vi "getGoalByName.vi"(7 "Category Name":string, 8 "error in (no error)":errorcluster, 9 "Month":T1, 10 "YYYY":i32, 11 "Account History in":refnum<class "Account History.lvclass">) -> (0 "error out":errorcluster, 2 "Goal":refnum<class "Goal.lvclass">, 3 "Account History out":refnum<class "Account History.lvclass">)   [LabVIEW 2018, in "Account History.lvclass"]
uses:
  Account History.lvclass
  Month.ctl
  Goal/Goal.lvclass
  Category/Category.lvclass
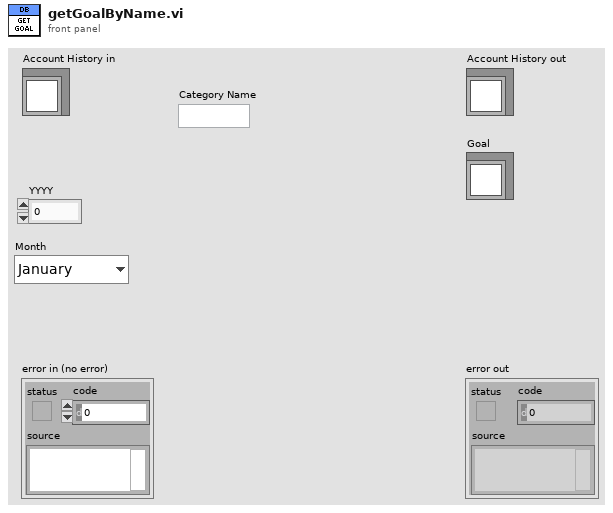
[diagram p1: front panel]
types:
  T1 = typedef "Account History.lvclass/Month.ctl" = enum16{"January", "February", "March", "April", "May", "June", "July", "August", "September", "October", "November", "December"}
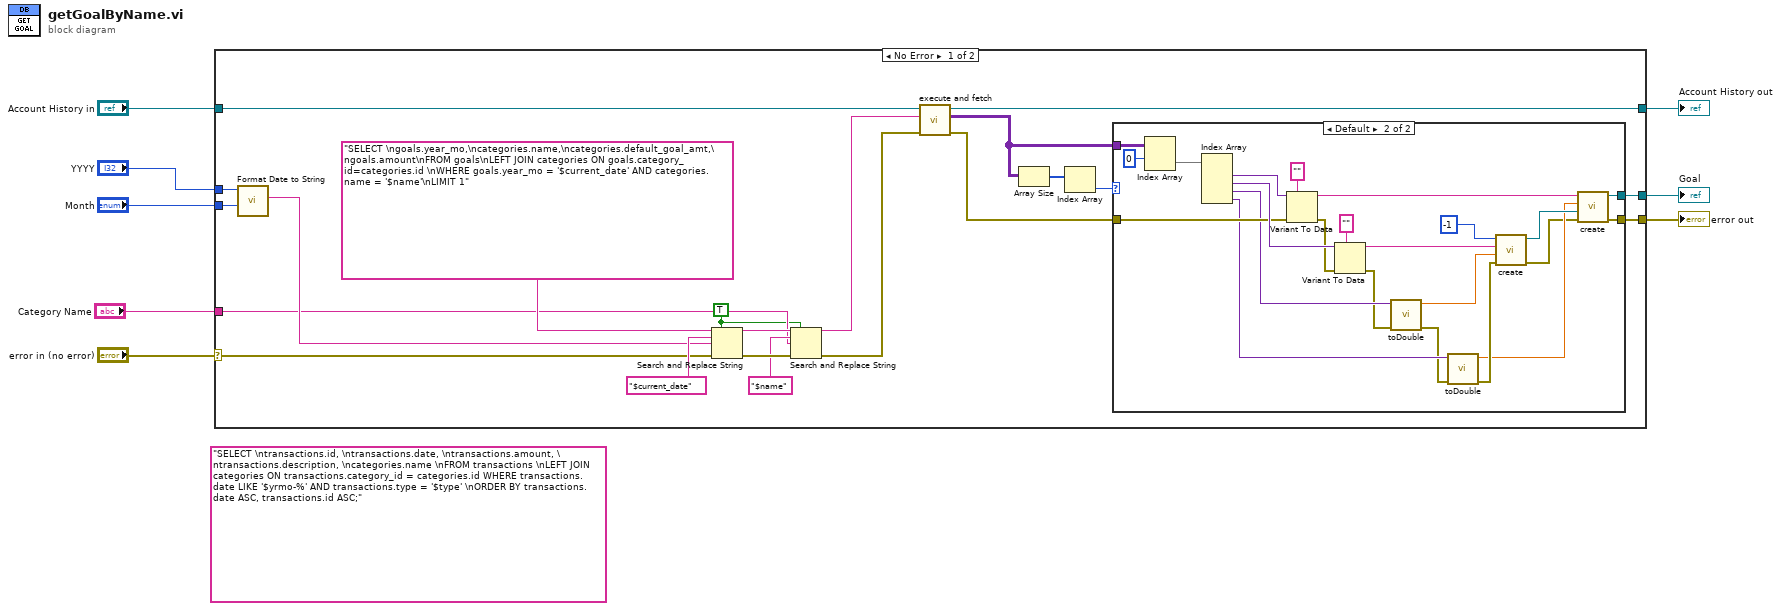
[diagram p0: block diagram]
diagram:
  (unwired) "SELECT \ntransactions.id, \ntransactions.date, \ntransactions.amount, \ntransactions.description, \ncategories.name \nFROM transactions \nLEFT JOIN categories ON transactions.category_id = categories.id WHERE transactions.date LIKE '$yrmo-%' AND transactions.type = '$type' \nORDER BY transactions.date ASC, transactions.id ASC;"
  n1 = case shown="No Error" "error in (no error)" {
    selector: "error in (no error)" -> [w23 w55]
    tunnel: [w14 w55] -> w7
    tunnel: [w26 w54] -> w5
    tunnel: "Account History in" -> [w27 w54]
    tunnel: "YYYY" -> [w29 _]
    tunnel: "Month" -> [w28 _]
    tunnel: "Category Name" -> [w16 _]
    tunnel: [w13 _] -> w1
    frame No Error {
      w15 = TRUE ("replace all? (F)")
      n2 = call "Format Date to String.vi"("Month"=w28, "YYYY"=w29) -> ("Year-Mo"=w22:string)  [unwired: 9 in]
      n3 = Search and Replace String(replace all?=w15, input string="SELECT \ngoals.year_mo,\ncategories.name,\ncategories.default_goal_amt,\ngoals.amount\nFROM goals\nLEFT JOIN categories ON goals.category_id=categories.id \nWHERE goals.year_mo = '$current_date' AND categories.name = '$name'\nLIMIT 1", search string="$current_date", replace string=w22, error in=w23) -> (result string=w20:string, error out=w21:errorcluster)  [unwired: 3 in, 2 out]
      n4 = Search and Replace String(replace all?=w15, input string=w20, search string="$name", replace string=w16, error in=w21) -> (result string=w19:string, error out=w18:errorcluster)  [unwired: 3 in, 2 out]
      n5 = call "execute and fetch.vi"("error in (no error)"=w18, "SQL query"=w19, "Database in"=w27) -> ("error out"=w12:errorcluster, "recordset data"=w11:variant[][], "Database out"=w26:refnum<class "Account History.lvclass">)  [unwired: 5 in, 1 out]
      n6 = Array Size(array=w11) -> (size(s)=w10:i32[])
      n7 = Index Array(array=w10) -> (element=w9:i32)  [unwired: 1 in]
      n8 = case shown="Default" w9 {
        tunnel: [w30 w40] -> w14
        tunnel: [_ w39] -> w13
        tunnel: w12 -> [w30 w38]
        tunnel: w11 -> [_ w31]
        frame 0 {
        }
        frame Default {
          n9 = Index Array(array=w31, index (row)=0) -> (element=w53:variant[])  [unwired: 1 in]
          n10 = Index Array(array=w53) -> (element #1=w52:variant, element #2=w51:variant, element #3=w36:variant, element #4=w37:variant)  [unwired: 4 in]
          n11 = Variant To Data(error in=w38, type="", Variant=w52) -> (data=w49:string, error out=w45:errorcluster)
          n12 = Variant To Data(error in=w45, type="", Variant=w51) -> (data=w47:string, error out=w35:errorcluster)
          n13 = call "toDouble.vi"("error in (no error)"=w35, "Value"=w36) -> ("error out"=w33:errorcluster, "type"=w34:dbl)  [unwired: 8 in]
          n14 = call "toDouble.vi"("error in (no error)"=w33, "Value"=w37) -> ("error out"=w44:errorcluster, "type"=w42:dbl)  [unwired: 8 in]
          n15 = call "create.vi"("error in (no error)"=w44, "Default Goal Amount"=w34, "Name"=w47, "id"=-1) -> ("error out"=w41:errorcluster, "Category out"=w43:refnum<class "Category.lvclass">)  [unwired: 6 in]
          n16 = call "create.vi"("error in (no error)"=w41, "Category.lvclass"=w43, "Amount"=w42, "Date"=w49) -> ("error out"=w40:errorcluster, "Goal out"=w39:refnum<class "Goal.lvclass">)  [unwired: 6 in]
        }
      }
    }
    frame Error {
    }
  }
  "error out" <- w7
  "Account History out" <- w5
  "Goal" <- w1
